vi "SetHandlerLevel.vi"(8 "error in (no error)":errorcluster, 10 "Level":T1=enum."WARNING", 11 "Handler in":refnum<class "Handler.lvclass">) -> (0 "error out":errorcluster, 3 "Handler out":refnum<class "Handler.lvclass">)   [LabVIEW 2022 SP3, in "Logger.lvlib" / "Handler.lvclass"]
uses:
  Handler.lvclass
  Handler.lvclass/Handler.ctl
  Logger/_Level.ctl
  Logger/Logger.lvclass
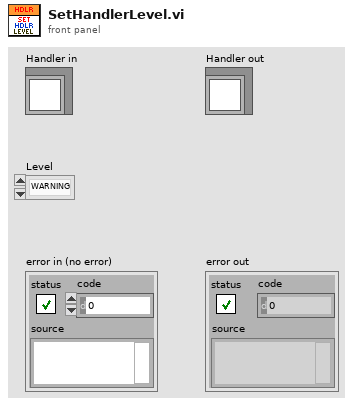
[diagram p1: front panel]
types:
  T1 = typedef "Logger.lvlib/Logger.lvclass/_Level.ctl" = enum16{"NOTSET", "DEBUG", "INFO", "WARNING", "ERROR", "CRITICAL"}
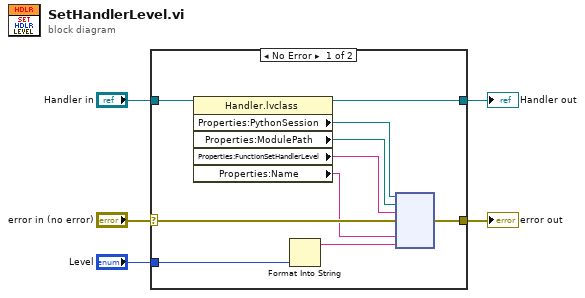
[diagram p0: block diagram]
diagram:
  n1 = case shown="No Error" "error in (no error)" {
    selector: "error in (no error)" -> [w15 w16]
    tunnel: [w14 w16] -> w4
    tunnel: "Level" -> [w13 _]
    tunnel: "Handler in" -> [w11 _]
    tunnel: [w9 _] -> w1
    frame No Error {
      n2 = property class="Handler.lvclass"(reference=w11) -> (reference out=w9:refnum<class "Handler.lvclass">, "Properties:PythonSession"=w6:refnum<k35>, "Properties:ModulePath"=w7:path, "Properties:FunctionSetHandlerLevel"=w8:string, "Properties:Name"=w10:string)  [unwired: 1 in, 1 out]
      n3 = Format Into String(w13) -> (resulting string=w12:string)  [unwired: 3 in, 1 out]
      n4 = node(w6, w7, w8, w15, w10, w12) -> (w14:errorcluster)  [unwired: 4 in, 3 out]
    }
    frame Error {
    }
  }
  "error out" <- w4
  "Handler out" <- w1
